vi "Add Frame.vi"(8 "error in (no error)":errorcluster, 11 "Node Ptr":u64 format="%.0x") -> (0 "error out":errorcluster)   [LabVIEW 2024, in "Diagnostics Addon System Explorer.lvlib"]
uses:
  Diagnostics Addon System Explorer.lvlib
  Types/Frame.Export.ctl
  Addon Shared/Types/Signal.ctl
  Addon Shared/SubVIs/Constants.vi
  <vilib>/NI VeriStand/Custom Device API/NI VeriStand - Get Item Parent.vi
  <vilib>/NI VeriStand/Custom Device API/Custom Device API.lvlib
  <vilib>/NI VeriStand/Custom Device Tools/Custom Device Utility Library/Custom Device Utility Library.lvlib
  Addon Shared/Diagnostics Addon Shared.lvlib
panel:
  in  "Tag":string
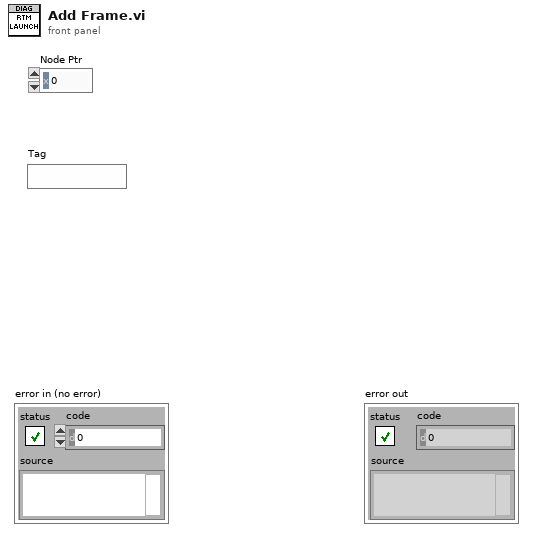
[diagram p1: front panel]
types:
  T1 = typedef "Diagnostics Addon Shared.lvlib/Type.ctl" = enum16{"DID", "CDID", "PID", "CPID", "Read Memory", "Write Memory", "IO Control", "Routine Start", "Routine Request", "Routine Stop", "User Defined", "DTC Control", "Clear DTCs", "Read DTCs", "Start DTCs", "DTC Change Count", "Tester Present", "Unlock ECU", "Reset ECU", "Diag Session Control", "Communication Control", "DPID Control", "Poll Control", "Diag Comm Port Control"}
  T2 = typedef "Custom Device API.lvlib/Custom Device Item Ref.ctl" = u64
  T3 = typedef "Custom Device API.lvlib/Custom Device Item Info.ctl" = cluster{"Name":string, "Is Channel":bool, "GUID":string, "Is Waveform":bool}
  T4 = typedef "Diagnostics Addon Shared.lvlib/Signal.ctl" = cluster{"Start Bit":u32, "Length":u32, "Scaling Factor":dbl, "Scaling Offset":dbl, "Minimum":dbl, "Maximum":dbl, "Data Type":u32, "Byte Order":u32, "Default Value":dbl, "Name":string, "Units":string}
  T5 = typedef "Diagnostics Addon System Explorer.lvlib/Frame.Export.ctl" = cluster{"Name":string, "ID":u32, "Signals":T4[]}
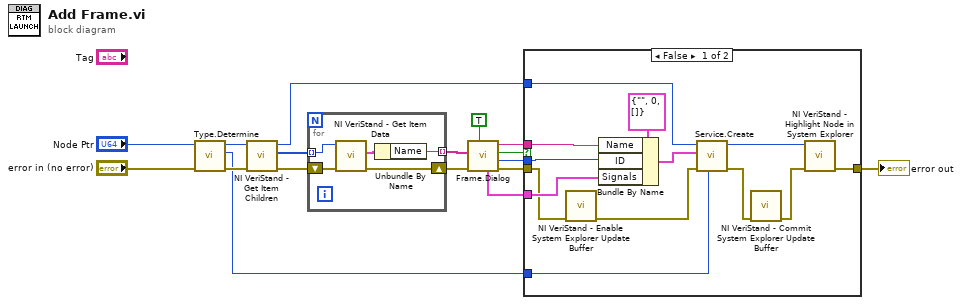
[diagram p0: block diagram]
diagram:
  n1 = call "Type.Determine.vi"("error in (no error)"="error in (no error)", "Node Ptr"="Node Ptr") -> ("error out"=w8:errorcluster, "Type"=w3:T1, "Item Ref out"=w7:T2)  [unwired: 6 in, 1 out]
  n2 = call <vilib>:"NI VeriStand - Get Item Children.vi"("error in (no error)"=w8, "Item Ref in"=w7) -> ("error out"=w17:errorcluster, "Child Refs"=w10:T2[], "Item Ref out"=w9:T2)  [unwired: 6 in, 1 out]
  n3 = for {
    tunnel: [w20] -> w16 mode=indexing
    shift-right: [w19] -> w15
    shift-left: w17 -> [w21]
    tunnel: w10 -> [w18] mode=indexing
    n4 = call <vilib>:"NI VeriStand - Get Item Data.vi"("error in (no error)"=w21, "Item Ref in"=w18) -> ("error out"=w19:errorcluster, "Item Info"=w22:T3)  [unwired: 8 out]
    n5 = Unbundle By Name(w22) -> ("Name"=w20:string)
  }
  n6 = call "Frame.Dialog.vi"("Show Name&ID"=TRUE, "error in (no error)"=w15, "Existing PIDs"=w16) -> ("error out"=w13:errorcluster, "ID out"=w6:u16, "Cancel PID?"=w14:bool, "Name out"=w12:string, "Signals out"=w5:T4[])  [unwired: 4 in]
  n7 = case shown="False" w14 {
    tunnel: w13 -> [w29 w36]
    tunnel: w9 -> [w26 _]
    tunnel: w12 -> [w34 _]
    tunnel: [w35 w36] -> w11
    tunnel: w6 -> [w33 _]
    tunnel: w5 -> [w30 _]
    tunnel: w3 -> [w28 _]
    frame False {
      n8 = call <vilib>:"NI VeriStand - Enable System Explorer Update Buffer.vi"("error in (no error)"=w29) -> ("error out"=w24:errorcluster)  [unwired: 10 in]
      n9 = Bundle By Name(cluster=T5 {"Name"="", "ID"=0, "Signals"=[]} ("DIDPID"), "Name"=w34, "ID"=w33, "Signals"=w30) -> (w27:T5)
      n10 = call "Service.Create.vi"("Type"=w28, "error in (no error)"=w24, "Variant"=w27, "Section Ptr"=w26) -> ("error out"=w23:errorcluster, "Parent Ref out"=w25:T2)  [unwired: 6 in]
      n11 = call <vilib>:"NI VeriStand - Commit System Explorer Update Buffer.vi"("error in (no error)"=w23) -> ("error out"=w31:errorcluster)  [unwired: 10 in]
      n12 = call <vilib>:"NI VeriStand - Highlight Node in System Explorer.vi"("error in (no error)"=w31, "Item Ref in"=w25) -> ("error out"=w35:errorcluster)  [unwired: 8 in, 1 out]
    }
    frame True {
    }
  }
  "error out" <- w11
